vi "Find Connection Route.vi"(8 "error in (no error)":errorcluster, 9 "channel 2":string, 10 "channel 1":string, 11 "Route Manager in":refnum<class "Route Manager.lvclass">) -> (0 "error out":errorcluster, 1 "relays to close":i32[](array[numeric]), 2 "relays to open":i32[](array[numeric]), 3 "Route Manager out":refnum<class "Route Manager.lvclass">)   [LabVIEW 2015, in "Route Manager.lvclass"]
uses:
  Route Manager.lvclass
  Route Manager.lvclass/Route Manager.ctl
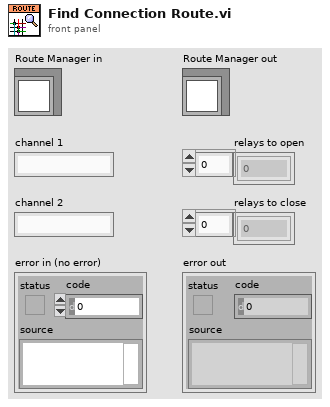
[diagram p1: front panel]
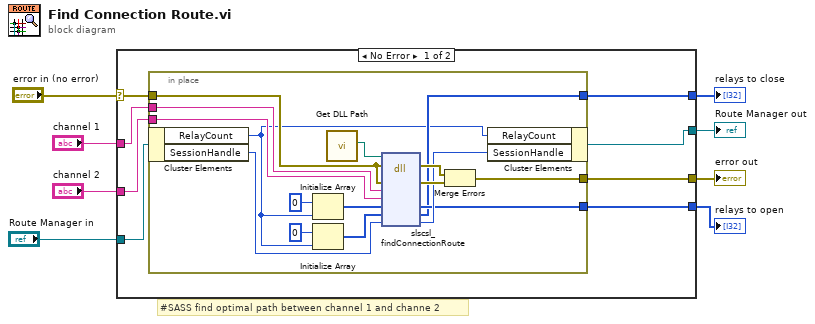
[diagram p0: block diagram]
diagram:
  # "#SASS find optimal path between channel 1 and channe 2"
  n1 = case shown="No Error" "error in (no error)" {
    selector: "error in (no error)" -> [w16 w34]
    tunnel: [w15 w34] -> w7
    tunnel: [w13 w33] -> w5
    tunnel: "Route Manager in" -> [w14 w33]
    tunnel: [w9 _] -> w4
    tunnel: [w10 _] -> w3
    tunnel: "channel 1" -> [w12 _]
    tunnel: "channel 2" -> [w11 _]
    frame No Error {
      n2 = in-place {
        in-place-border: w16 -> [w22]
        in-place-border: [w29] -> w15
        in-place-border: [w26] -> w9
        in-place-border: [w25] -> w10
        in-place-border: w12 -> [w24]
        in-place-border: w11 -> [w23]
        n3 = in-place-cluster #1(w14) -> ("RelayCount"=w17:i32, "SessionHandle"=w28:u64)
        n4 = Initialize Array(0 ("element"), w17) -> (w19:i32[])
        n5 = Initialize Array(0 ("element"), w17) -> (w18:i32[])
        n6 = call "Get DLL Path.vi"() -> ("slscsl DLL Path"=w31:path)  [unwired: 11 in]
        n7 = dll-call lib="?" fn="slscsl_findConnectionRoute"(path in=w31, error in=w22, "errorCluster"=w22, "ch1"=w24, "ch2"=w23, "openList"=w19, "closeList"=w18, "sessionHandle"=w28) -> (error out=w32:errorcluster, "errorCluster"=w30:errorcluster, "openList"=w26:i32[], "closeList"=w25:i32[], "sessionHandle"=w27:u64)  [unwired: 4 in, 1 out]
        n8 = Merge Errors(w32, w30) -> (w29:errorcluster)
        n9 = in-place-cluster #1("RelayCount"=w17, "SessionHandle"=w27) -> (w13:refnum<class "Route Manager.lvclass">)
      }
    }
    frame Error {
    }
  }
  "error out" <- w7
  "relays to open" <- w4
  "relays to close" <- w3
  "Route Manager out" <- w5
